vi "ex1_snap Color.vi"() -> ()   [LabVIEW 2010]
panel:
  in  "NumColorPanes":u32=1
  in  "stop":bool
  out "Image":T1(plugin-control)
  in  "Blue Exposure":dbl=10.0
  in  "Red Exposure":dbl=10.0
  in  "Green Exposure":dbl=10.0
  out "error status":errorcluster
  # "msec"
  # "msec"
  # "msec"
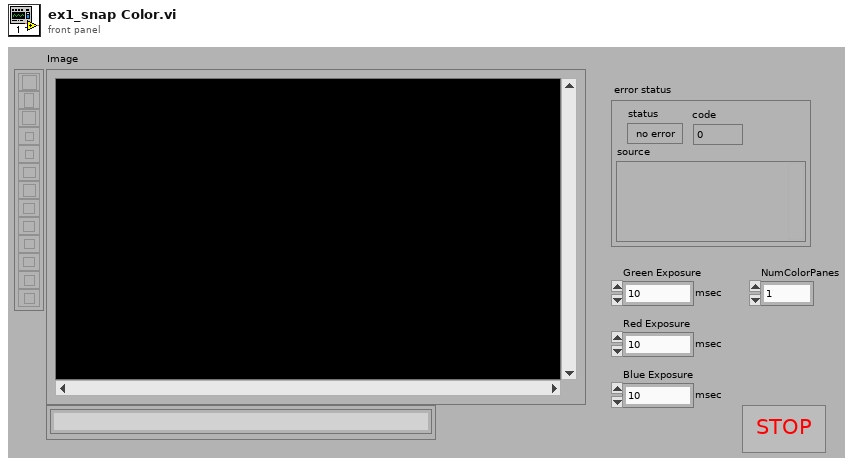
[diagram p1: front panel]
types:
  T1 = typedef "IMAQ Image.ctl" = refnum<image>
  T2 = typedef "Image Type" = u32
  T3 = cluster{"Green Exposure":dbl, "Red Exposure":dbl, "Blue Exposure":dbl}
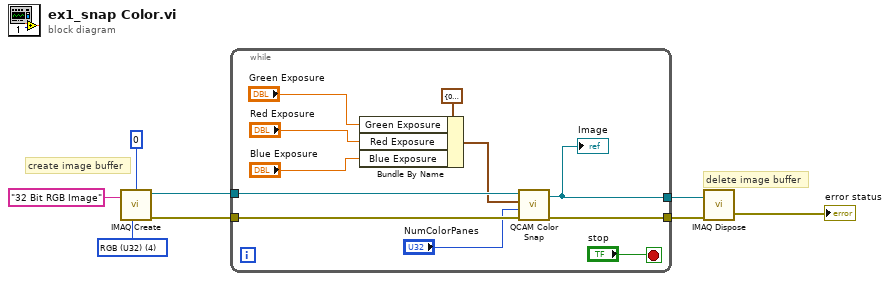
[diagram p0: block diagram]
diagram:
  w1 = T2 4 items=["Grayscale (U8)", "Grayscale (I16)", "Grayscale (SGL)", "Complex (CSG)", "RGB (U32)", "HSL (U32)", "RGB (U64)", "Grayscale (U16)"] ("Image Type")
  # "create image buffer"
  # "delete image buffer"
  n1 = call "IMAQ Create"("Border Size"=0, "Image Name"="32 Bit RGB Image", "Image Type"=w1) -> ("New Image"=w7:T1, "error out"=w6:errorcluster)  [unwired: 1 in, 1 out]
  n2 = while {
    tunnel: w7 -> [w19]
    tunnel: w6 -> [w18]
    tunnel: [w12] -> w3
    tunnel: [w11] -> w2
    stop <- "stop" stop-if-true
    n3 = Bundle By Name(cluster=T3 {"Green Exposure"=0.0, "Red Exposure"=0.0, "Blue Exposure"=0.0} ("Exposures"), "Green Exposure"="Green Exposure", "Red Exposure"="Red Exposure", "Blue Exposure"="Blue Exposure") -> (w13:T3)
    n4 = call <userlib>:"QCAM Color Snap.vi"("error in (no error)"=w18, "NumColorPanes"="NumColorPanes", "Exposures"=w13, "New Image"=w19) -> ("error out"=w11:errorcluster, "Image Out"=w12:T1)  [unwired: 2 in, 4 out]
    "Image" <- w12
  }
  n5 = call "IMAQ Dispose"("Image"=w3, "error in (no error)"=w2) -> ("error out"=→"error status":errorcluster)  [unwired: 1 in, 3 out]
